vi "Stamp Version.vi"(8 "error in (no error)":errorcluster, 11 "Serial port":refnum<visa-resource-name>) -> (0 "error out":errorcluster, 1 "success":bool, 2 "version":string, 3 "Serial port out":refnum<visa-resource-name>)   [LabVIEW 2010]
panel:
  out "x-y":u32
  in  "versions":string="AB"
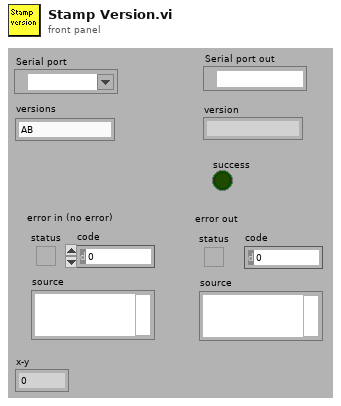
[diagram p1: front panel]
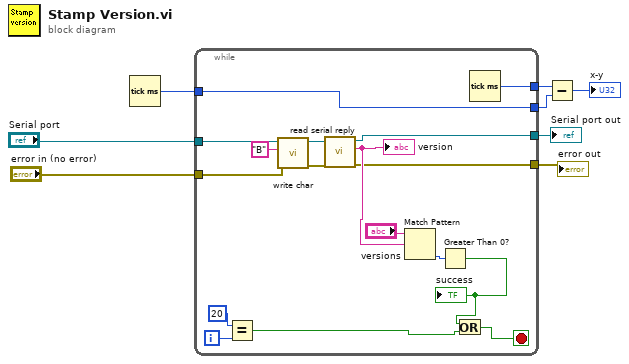
[diagram p0: block diagram]
diagram:
  n1 = Tick Count (ms)() -> (millisecond timer value=w2:u32)
  n2 = while {
    tunnel: [w24] -> w8
    tunnel: "Serial port" -> [w23]
    tunnel: [w17] -> w6
    tunnel: "error in (no error)" -> [w16]
    tunnel: [w10] -> w4
    tunnel: [w9] -> w3
    tunnel: w2 -> [w9]
    i -> [w15]
    stop <- w11 stop-if-true
    n3 = Equal?(x=20, y=w15) -> (x = y?=w12:bool)
    n4 = call "write char.vi"("error in (no error)"=w16, "write buffer"="B", "Serial port"=w23) -> ("error out"=w21:errorcluster, "Serial Port"=w25:refnum<visa-resource-name>)  [unwired: 6 in, 1 out]
    n5 = call "read serial reply.vi"("error in (no error)"=w21, "Serial Port"=w25) -> ("error out"=w17:errorcluster, "reply"=w19:string, "Serial Port out"=w24:refnum<visa-resource-name>)  [unwired: 7 in]
    "version" <- w19
    n6 = Match Pattern(string="versions", regular expression=w19) -> (offset past match=w18:i32)  [unwired: 1 in, 3 out]
    n7 = Greater Than 0?(x=w18) -> (x > 0?=w13:bool)
    "success" <- w13
    n8 = Or(x=w13, y=w12) -> (x .or. y?=w11:bool)
    n9 = Tick Count (ms)() -> (millisecond timer value=w10:u32)
  }
  "Serial port out" <- w8
  "error out" <- w6
  n10 = Subtract(x=w4, y=w3) -> (x-y=→"x-y":u32)
